vi "Read INI.vi"(0 "Path":path, 1 "error in (no error)":errorcluster) -> (2 "Current Calibration":dbl[][](array[numeric]), 3 "Voltage Calibration":dbl[][](array[numeric]), 4 "error out":errorcluster)   [LabVIEW 2022 SP3]
uses:
  <vilib>/Utility/config.llb/Read Key (Double).vi
  <vilib>/Utility/config.llb/NI_LVConfig.lvlib
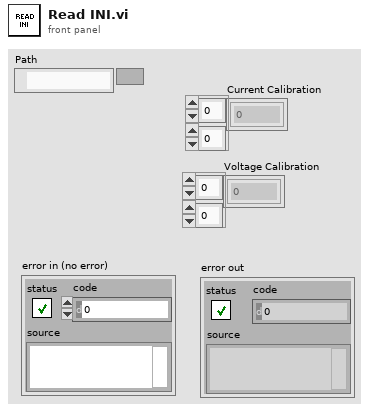
[diagram p1: front panel]
types:
  T1 = typedef "NI_LVConfig.lvlib/Config Data RefNum.ctl" = refnum<k1>
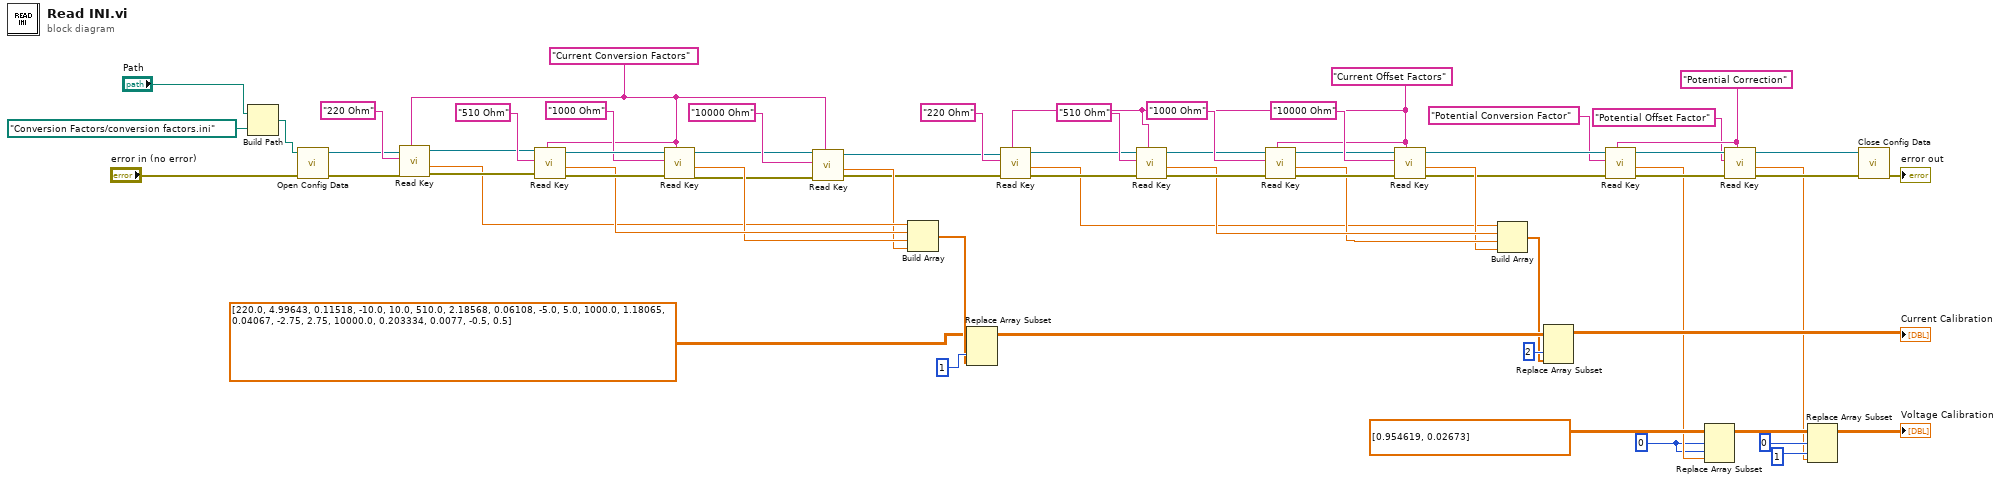
[diagram p0: block diagram]
diagram:
  w6 = 0 ("disabled index (row)")
  w13 = "Current Offset Factors" ("section")
  w11 = "Potential Correction" ("section")
  w12 = "Current Conversion Factors" ("section")
  n1 = Build Path(base path="Path", name or relative path=path "Conversion Factors/conversion factors.ini") -> (appended path=w57:path)
  n2 = call <vilib>:"Open Config Data.vi"("error in (no error)"="error in (no error)", "configuration file path"=w57) -> ("error out"=w33:errorcluster, "refnum"=w32:T1)  [unwired: 7 in, 1 out]
  n3 = call-poly <vilib>:"Read Key.vi"("section"=w12, "error in (no error)"=w33, "key"="220 Ohm", "refnum"=w32) -> ("error out"=w34:errorcluster, "value"=w31:dbl, "refnum out"=w35:T1)  [unwired: 4 in, 1 out]
  n4 = call-poly <vilib>:"Read Key.vi"("section"=w12, "error in (no error)"=w34, "key"="510 Ohm", "refnum"=w35) -> ("error out"=w61:errorcluster, "value"=w53:dbl, "refnum out"=w63:T1)  [unwired: 4 in, 1 out]
  n5 = call-poly <vilib>:"Read Key.vi"("section"=w12, "error in (no error)"=w61, "key"="1000 Ohm", "refnum"=w63) -> ("error out"=w20:errorcluster, "value"=w52:dbl, "refnum out"=w23:T1)  [unwired: 4 in, 1 out]
  n6 = call-poly <vilib>:"Read Key.vi"("section"=w12, "error in (no error)"=w20, "key"="10000 Ohm", "refnum"=w23) -> ("error out"=w21:errorcluster, "value"=w24:dbl, "refnum out"=w22:T1)  [unwired: 4 in, 1 out]
  n7 = Build Array(w31, w53, w52, w24) -> (w51:dbl[])
  n8 = Replace Array Subset(array=dbl[][] [[220.0, 4.99643, 0.11518, -10.0, 10.0], [510.0, 2.18568, 0.06108, -5.0, 5.0], [1000.0, 1.18065, 0.04067, -2.75, 2.75], [10000.0, 0.203334, 0.0077, -0.5, 0.5]] ("Conversion and Correction"), new element=w51, index (col)=1 ("disabled index (col)")) -> (w39:dbl[][])  [unwired: 1 in]
  n9 = call-poly <vilib>:"Read Key.vi"("section"=w13, "error in (no error)"=w21, "key"="220 Ohm", "refnum"=w22) -> ("error out"=w28:errorcluster, "value"=w27:dbl, "refnum out"=w29:T1)  [unwired: 4 in, 1 out]
  n10 = call-poly <vilib>:"Read Key.vi"("section"=w13, "error in (no error)"=w28, "key"="510 Ohm", "refnum"=w29) -> ("error out"=w46:errorcluster, "value"=w43:dbl, "refnum out"=w44:T1)  [unwired: 4 in, 1 out]
  n11 = call-poly <vilib>:"Read Key.vi"("section"=w13, "error in (no error)"=w46, "key"="1000 Ohm", "refnum"=w44) -> ("error out"=w47:errorcluster, "value"=w42:dbl, "refnum out"=w45:T1)  [unwired: 4 in, 1 out]
  n12 = call-poly <vilib>:"Read Key.vi"("section"=w13, "error in (no error)"=w47, "key"="10000 Ohm", "refnum"=w45) -> ("error out"=w14:errorcluster, "value"=w41:dbl, "refnum out"=w19:T1)  [unwired: 4 in, 1 out]
  n13 = Build Array(w27, w43, w42, w41) -> (w38:dbl[])
  n14 = Replace Array Subset(array=w39, new element=w38, index (col)=2) -> (→"Current Calibration":dbl[][])  [unwired: 1 in]
  n15 = call-poly <vilib>:"Read Key.vi"("section"=w11, "error in (no error)"=w14, "key"="Potential Conversion Factor", "refnum"=w19) -> ("error out"=w15:errorcluster, "value"=w7:dbl, "refnum out"=w18:T1)  [unwired: 4 in, 1 out]
  n16 = Replace Array Subset(array=dbl[][] [[0.954619, 0.02673]] ("Conversion and Correction"), new element=w7, index (row)=w6, index (col)=w6) -> (w5:dbl[][])
  n17 = call-poly <vilib>:"Read Key.vi"("section"=w11, "error in (no error)"=w15, "key"="Potential Offset Factor", "refnum"=w18) -> ("error out"=w16:errorcluster, "value"=w2:dbl, "refnum out"=w17:T1)  [unwired: 4 in, 1 out]
  n18 = Replace Array Subset(array=w5, new element=w2, index (row)=0, index (col)=1 ("disabled index (col)")) -> (→"Voltage Calibration":dbl[][])
  n19 = call <vilib>:"Close Config Data.vi"("error in (no error)"=w16, "refnum"=w17) -> ("error out"=→"error out":errorcluster)  [unwired: 8 in, 1 out]
